vi "take imge.vi"() -> ()   [LabVIEW 2019]
uses:
  <vilib>/vision/Image Controls.llb/IMAQ Image.ctl
panel:
  out "Image Out (duplicate)":T1
  out "Image Out":T1(plugin-control)
  out "Frame Rate":dbl
  in  "Boolean":bool
  in  "Stop (F)":bool
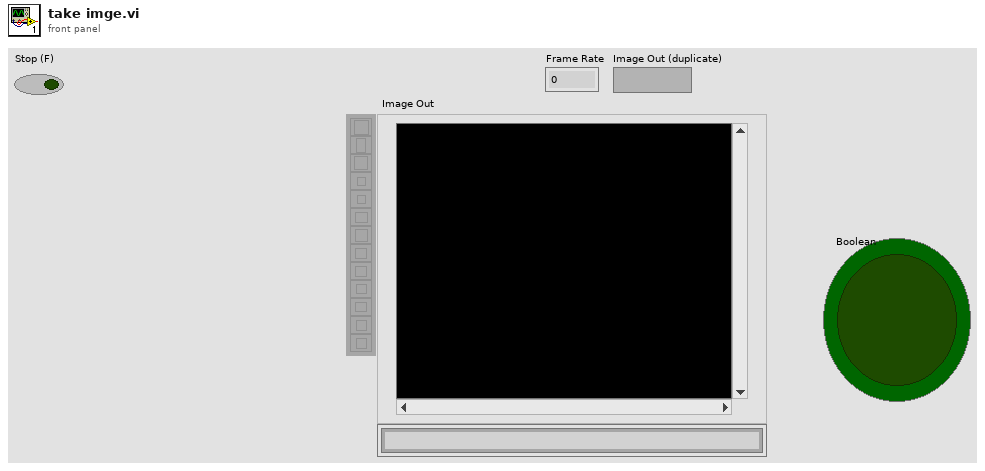
[diagram p1: front panel]
types:
  T1 = typedef "IMAQ Image.ctl" = refnum<image>
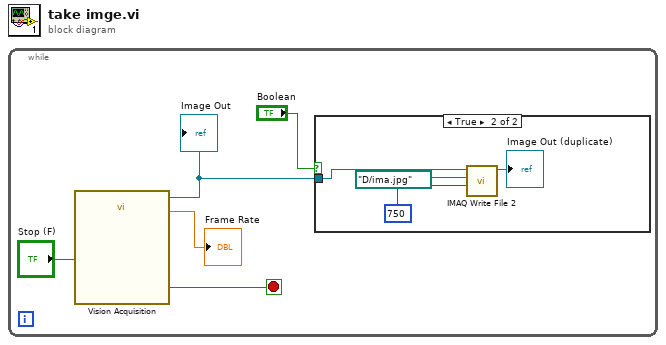
[diagram p0: block diagram]
diagram:
  n1 = while {
    stop <- w4 stop-if-true
    n2 = call "Vision Acquisition"("Stop (F)"="Stop (F)") -> ("Image Out"=w2:T1, "Frame Rate"=→"Frame Rate":dbl, "Stopped"=w4:bool)  [unwired: 23 in, 1 out]
    "Image Out" <- w2
    n3 = case shown="True" "Boolean" {
      tunnel: w2 -> [_ w8]
      frame False {
      }
      frame True {
        n4 = call-poly "IMAQ Write File 2"("Image Quality"=u32 750, "File Path"=path "D:/ima.jpg", "Image"=w8) -> ("Image Out (duplicate)"=→"Image Out (duplicate)":T1)  [unwired: 7 in, 1 out]
      }
    }
  }
